vi "Create Evaluations.vi"(8 "error in (no error)":errorcluster, 11 "CDMA2K_SEM in":refnum<class "CDMA2K_SEM.lvclass">) -> (0 "error out":errorcluster, 2 "Evaluations Out":T1[](array[typedef]) {"Low Limit" format="%#_13g"; "SI Scaling" items=["femto"=-15, "pico"=-12, "nano"=-9, "micro"=-6, "milli"=-3, "percent"=-2, ""=0, "kilo"=3, "mega"=6, "giga"=9, "tera"=12]}, 3 "CDMA2K_SEM out":refnum<class "CDMA2K_SEM.lvclass">)   [LabVIEW 2016, in "SeqAuto Evaluations.lvlib" / "CDMA2K_SEM.lvclass"]
uses:
  CDMA2K_SEM.lvclass
  C:/projects/STS/Common/Sequence Automation/Plugins/SeqAuto IEvaluation.lvlibp/SeqAuto IEvaluation.lvclass
  Plugins/TestStand API Tools (TSAT).lvlibp/Evaluation Actions/Includes/Controls/TSAT Evaluation.ctl
  Plugins/TestStand API Tools (TSAT).lvlibp/Evaluation Actions/Includes/Controls/TSAT Eval SI Unit Scaling.ctl
  Plugins/TestStand API Tools (TSAT).lvlibp/Evaluation Actions/Includes/Controls/TSAT Evaluation Type.ctl
  Plugins/SeqAuto IEvaluation.lvlibp/Read Measurement Name.vi
  Plugins/TestStand API Tools (TSAT).lvlibp/Evaluation Actions/TSAT Evaluation Actions.lvlib
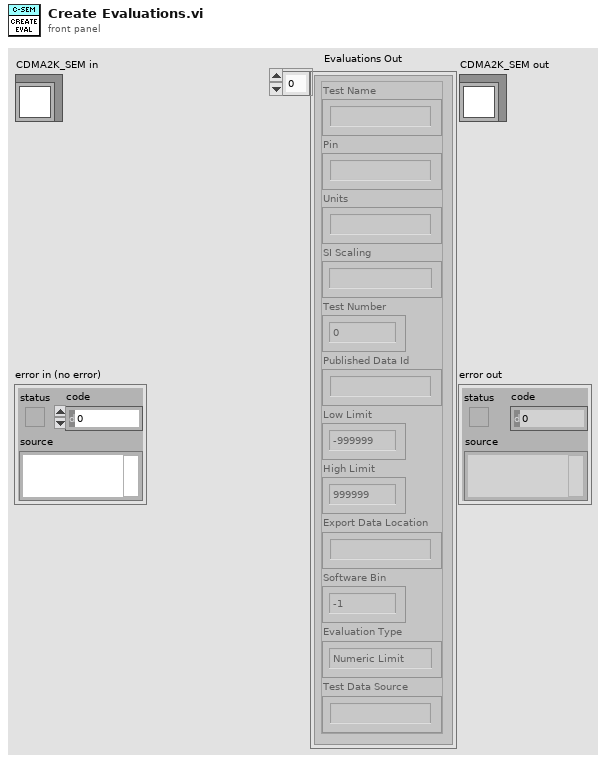
[diagram p1: front panel]
types:
  T1 = typedef "TestStand API Tools (TSAT).lvlibp/TSAT Evaluation Actions.lvlib/TSAT Evaluation.ctl" = cluster{"Test Name":string, "Pin":string, "Units":string, "SI Scaling":T2, "Test Number":i32, "Published Data Id":string, "Low Limit":dbl, "High Limit":dbl, "Export Data Location":string, "Software Bin":i64, "Evaluation Type":T3, "Test Data Source":string}
  T2 = typedef "TestStand API Tools (TSAT).lvlibp/TSAT Evaluation Actions.lvlib/TSAT Eval SI Unit Scaling.ctl" = i16
  T3 = typedef "TestStand API Tools (TSAT).lvlibp/TSAT Evaluation Actions.lvlib/TSAT Evaluation Type.ctl" = enum16{"Numeric Limit", "Pass/Fail", "None"}
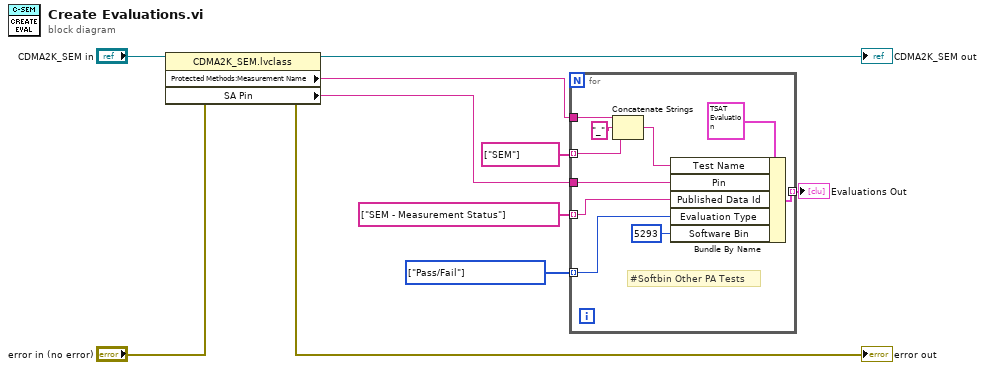
[diagram p0: block diagram]
diagram:
  w2 = T3[] [enum."Pass/Fail"] items=["Numeric Limit", "Pass/Fail", "None"]
  n1 = property class="CDMA2K_SEM.lvclass"(reference="CDMA2K_SEM in", error in="error in (no error)") -> (reference out=→"CDMA2K_SEM out":refnum<class "CDMA2K_SEM.lvclass">, error out=→"error out":errorcluster, "Protected Methods:Measurement Name"=w6:string, "SA Pin"=w4:string)
  n2 = for {
    tunnel: w4 -> [w19]
    tunnel: w6 -> [w18]
    tunnel: string[] ["SEM"] -> [w17] mode=indexing
    tunnel: string[] ["SEM - Measurement Status"] -> [w14] mode=indexing
    tunnel: w2 -> [w13] mode=indexing
    tunnel: [w12] -> w1 mode=indexing
    # "#Softbin Other PA Tests"
    n3 = Concatenate Strings(w18, "_" ("string"), w17) -> (w16:string)
    n4 = Bundle By Name(cluster=T1 {"Test Name"="", "Pin"="", "Units"="", "SI Scaling"=0, "Test Number"=0, "Published Data Id"="", "Low Limit"=-999999.0, "High Limit"=999999.0, "Export Data Location"="", "Software Bin"=-1, "Evaluation Type"=enum."Numeric Limit", "Test Data Source"=""} ("Evaluation"), "Test Name"=w16, "Pin"=w19, "Published Data Id"=w14, "Evaluation Type"=w13, "Software Bin"=i64 5293) -> (w12:T1)
  }
  "Evaluations Out" <- w1
